vi "SVFA Magnitude and Phase to Real and Imaginary (NxM).vi"(0 "magnitude spectra":T10(array[cluster]), 2 "phase spectra":cluster{"x0":dbl, "dx":dbl, "phase":dbl[]}[][](array[cluster]), 4 "spectrum info in":T1[][](array[typedef]) {"x-axis units" items=["Time (s)"=0, "Frequency-CB (Hz)"=1, "Frequency-CPB (Hz)"=1248, "Frequency-Arbitrary (Hz)"=2357, "Quefrency (s)"=2, "Revolutions (rev)"=3, "Order"=4, "Speed (RPM)"=11, "Speed (rad/s)"=21, "Index"=65535]; "weighting filter" items=["Linear", "A-weighting", "B-weighting", "C-weighting", "ITU-R 468-4", "Dolby", "CCITT", "C-message", "Wb", "Wc", "Wd", "We", "Wf", "Wh", "Wj", "Wk", "Wm", "AES17 20 kHz lowpass", "AES17 40 kHz lowpass", "AES17 20 kHz highpass", "AES17 40 kHz highpass"]; "dB reference [EU]" format="%.2f"; "engineering units" items=["custom..."=0, "V"=1, "A"=21, "C"=30, "pC"=31, "s"=32, "-"=29, "Pa"=2, "N"=20, "g"=3, "m/s^2"=4, "m/s"=5, "m"=6, "mm/s"=12, "mm"=13, "micron/s"=14, "micron"=15, "in/s^2"=7, "in/s"=8, "in"=9, "mil/s"=10, "mil"=11, "rad/s^2"=16, "rad/s"=17, "rad"=18, "deg/s^2"=26, "deg/s"=27, "deg"=28, "RPM"=22, "cycle/s^2"=23, "Hz"=24, "cycle"=25, "strain"=19]; "spectral info"."window" items=["None "=0, "Hanning"=1, "Hamming"=2, "Blackman-Harris"=3, "Exact Blackman"=4, "Blackman"=5, "Flat Top"=6, "4 Term B-Harris "=7, "7 Term B-Harris"=8, "Low Sidelobe"=9, "Force - Exponential"=10, "Gaussian"=62]}, 5 "error in (no error)":errorcluster) -> (12 "Nyquist plots":T9(array[cluster]), 14 "real spectra":T8(array[cluster]), 16 "imaginary spectra":T7(array[cluster]), 17 "unit labels":string[][](array[string]), 18 "spectrum info out":T1[][](array[typedef]) {"x-axis units" items=["Time (s)"=0, "Frequency-CB (Hz)"=1, "Frequency-CPB (Hz)"=1248, "Frequency-Arbitrary (Hz)"=2357, "Quefrency (s)"=2, "Revolutions (rev)"=3, "Order"=4, "Speed (RPM)"=11, "Speed (rad/s)"=21, "Index"=65535]; "weighting filter" items=["Linear", "A-weighting", "B-weighting", "C-weighting", "ITU-R 468-4", "Dolby", "CCITT", "C-message", "Wb", "Wc", "Wd", "We", "Wf", "Wh", "Wj", "Wk", "Wm", "AES17 20 kHz lowpass", "AES17 40 kHz lowpass", "AES17 20 kHz highpass", "AES17 40 kHz highpass"]; "dB reference [EU]" format="%.2f"; "engineering units" items=["custom..."=0, "V"=1, "A"=21, "C"=30, "pC"=31, "s"=32, "-"=29, "Pa"=2, "N"=20, "g"=3, "m/s^2"=4, "m/s"=5, "m"=6, "mm/s"=12, "mm"=13, "micron/s"=14, "micron"=15, "in/s^2"=7, "in/s"=8, "in"=9, "mil/s"=10, "mil"=11, "rad/s^2"=16, "rad/s"=17, "rad"=18, "deg/s^2"=26, "deg/s"=27, "deg"=28, "RPM"=22, "cycle/s^2"=23, "Hz"=24, "cycle"=25, "strain"=19]; "spectral info"."window" items=["None "=0, "Hanning"=1, "Hamming"=2, "Blackman-Harris"=3, "Exact Blackman"=4, "Blackman"=5, "Flat Top"=6, "4 Term B-Harris "=7, "7 Term B-Harris"=8, "Low Sidelobe"=9, "Force - Exponential"=10, "Gaussian"=62]}, 19 "error out":errorcluster)   [LabVIEW 2017]
doc: "Converts spectra from polar components to rectangular components. This conversion can reduce the computational power necessary to view and process spectra. Wire data to the <B>magnitude spectrum</B> and <B>phase spectrum</B> inputs to determine the polymorphic instance to use or manually select the instance."
uses:
  <vilib>/addons/_NISVFA/_Shared subVIs/Controls/svc_Spectrum Info.ctl
  <vilib>/addons/_NISVFA/_Shared subVIs/Controls/svc_X-Axis Units.ctl
  <vilib>/addons/_NISVFA/_Shared subVIs/Controls/svc_Spectrum Type.ctl
  <vilib>/addons/_NISVFA/_Shared subVIs/Controls/svc_Engineering Units Text Ring.ctl
  <vilib>/addons/_NISVFA/_Shared subVIs/Controls/svc_Weighting Filter Text Ring.ctl
  <vilib>/addons/_NISVFA/_Shared subVIs/Controls/svc_Complimentary Spectrum Units.ctl
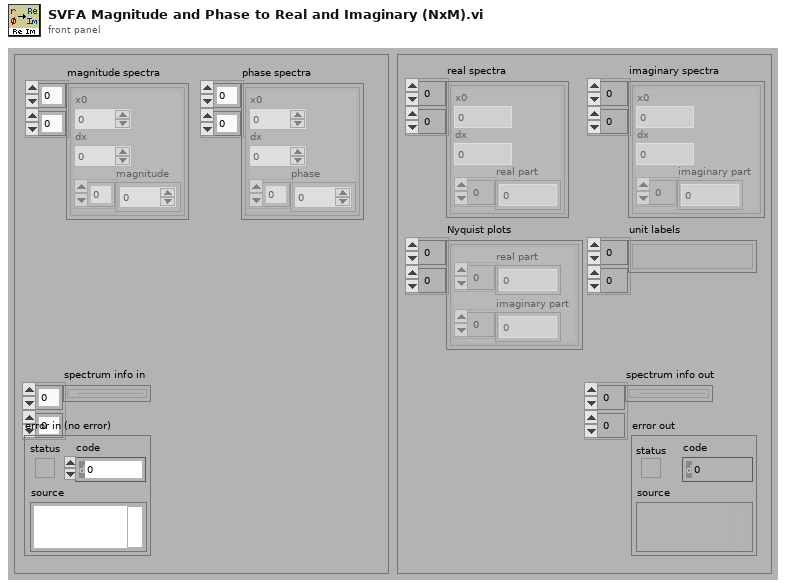
[diagram p1: front panel]
types:
  T1 = typedef "svc_Spectrum Info.ctl" = cluster{"channel name":string, "description":string, "x-axis units":T2, "spectral info":cluster{"spectrum type":T3, "linear/dB":enum16{"linear", "dB"}, "window":u16, "window size":i32, "FFT size":i32}, "engineering units":T4, "custom label":string, "dB reference [EU]":dbl, "peak units":enum16{"rms", "peak", "peak-peak"}, "weighting filter":T5, "spectral density?":bool, "unit label":string, "spectrum skewed?":bool, "complimentary spectrum units":T6}
  T2 = typedef "svc_X-Axis Units.ctl" = u16
  T3 = typedef "svc_Spectrum Type.ctl" = enum16{"FFT Spectrum [complex]", "Amplitude [Magnitude]", "Power [Magnitude^2]", "Cross Spectrum [complex]", "Frequency Response [Complex]"}
  T4 = typedef "svc_Engineering Units Text Ring.ctl" = u16
  T5 = typedef "svc_Weighting Filter Text Ring.ctl" = u16
  T6 = typedef "svc_Complimentary Spectrum Units.ctl" = enum16{"none", "radians", "degrees", "cycles", "imaginary"}
  T7 = cluster{"x0":dbl, "dx":dbl, "imaginary part":dbl[]}[][]
  T8 = cluster{"x0":dbl, "dx":dbl, "real part":dbl[]}[][]
  T9 = cluster{"real part":dbl[], "imaginary part":dbl[]}[][]
  T10 = cluster{"x0":dbl, "dx":dbl, "magnitude":dbl[]}[][]
  T11 = cluster{"real part":dbl[], "imaginary part":dbl[]}
  T12 = cluster{"x0":dbl, "dx":dbl, "imaginary part":dbl[]}
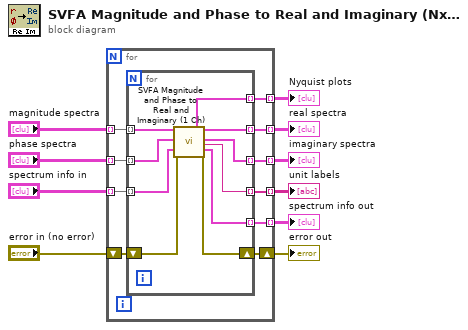
[diagram p0: block diagram]
diagram:
  n1 = for {
    tunnel: [w20] -> w10 mode=indexing
    tunnel: "magnitude spectra" -> [w19] mode=indexing
    tunnel: "phase spectra" -> [w18] mode=indexing
    tunnel: [w17] -> w7 mode=indexing
    tunnel: [w15] -> w5 mode=indexing
    tunnel: [w14] -> w4 mode=indexing
    tunnel: "spectrum info in" -> [w13] mode=indexing
    tunnel: [w12] -> w2 mode=indexing
    shift-right: [w16] -> w6
    shift-left: "error in (no error)" -> [w11]
    n2 = for {
      tunnel: [w23] -> w20 mode=indexing
      tunnel: w19 -> [w30] mode=indexing
      tunnel: w18 -> [w29] mode=indexing
      tunnel: [w24] -> w17 mode=indexing
      tunnel: [w22] -> w15 mode=indexing
      tunnel: [w21] -> w14 mode=indexing
      tunnel: w13 -> [w28] mode=indexing
      tunnel: [w25] -> w12 mode=indexing
      shift-right: [w26] -> w16
      shift-left: w11 -> [w27]
      n3 = call <vilib>:"SVFA Magnitude and Phase to Real and Imaginary (1 Ch).vi"("magnitude spectrum"=w30, "phase spectrum"=w29, "spectrum info in"=w28, "error in (no error)"=w27) -> ("Nyquist plot"=w23:T11, "real spectrum"=w24:cluster{"x0":dbl, "dx":dbl, "real part":dbl[]}, "imaginary spectrum"=w22:T12, "unit label"=w25:string, "spectrum info out"=w21:T1, "error out"=w26:errorcluster)  [unwired: 10 in]
    }
  }
  "Nyquist plots" <- w10
  "real spectra" <- w7
  "imaginary spectra" <- w5
  "error out" <- w6
  "spectrum info out" <- w4
  "unit labels" <- w2
